vi "Quaternion_Normalize.vi"(11 "Quaternion":T1={"R"=1.0, "V"=[0.0, 0.0, 0.0]}) -> (3 "Normalize":T1={"R"=1.0, "V"=[0.0, 0.0, 0.0]})   [LabVIEW 2019, in "Trajectory_Library.lvlib"]
doc: "Convenience constructors that takes in x and y values directly instead of having to construct a Translation2d.\n\nParameters:\n - X- The x component of the translational component of the pose.\n - Y - The y component of the translational component of the pose.\n - Rotation (Heading) - The rotational component of the pose.\n\nReturns:\n - OUT POSE - Output POSE"
uses:
  QUATERNION.ctl
  Trajectory_Library.lvlib
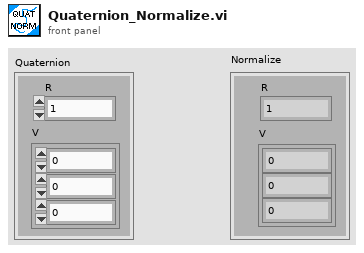
[diagram p1: front panel]
types:
  T1 = typedef "Trajectory_Library.lvlib/QUATERNION.ctl" = cluster{"R":dbl, "V":dbl[]}
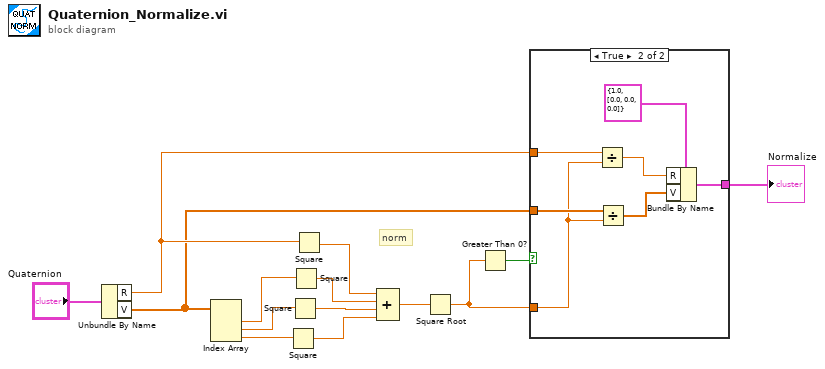
[diagram p0: block diagram]
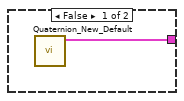
[diagram p2: hidden frame]
diagram:
  # "norm"
  n1 = Unbundle By Name("Quaternion") -> ("R"=w4:dbl, "V"=w3:dbl[])
  n2 = Index Array(array=w3) -> (element #1=w13:dbl, element #2=w12:dbl, element #3=w11:dbl)  [unwired: 3 in]
  n3 = Square(x=w11) -> (x^2=w8:dbl)
  n4 = Square(x=w12) -> (x^2=w9:dbl)
  n5 = Square(x=w13) -> (x^2=w10:dbl)
  n6 = Square(x=w4) -> (x^2=w6:dbl)
  n7 = Compound Arithmetic op=ADD(w6, w10, w9, w8) -> (w7:dbl)
  n8 = Square Root(x=w7) -> (sqrt(x)=w2:dbl)
  n9 = Greater Than 0?(x=w2) -> (x > 0?=w5:bool)
  n10 = case shown="True" w5 {
    tunnel: w4 -> [_ w22]
    tunnel: w3 -> [_ w21]
    tunnel: w2 -> [_ w20]
    tunnel: [w15 w16] -> w1
    frame False {
      n11 = call "Quaternion_New_Default.vi"() -> ("out Quaternion"=w15:T1)  [unwired: 11 in]
    }
    frame True {
      n12 = Divide(x=w22, y=w20) -> (x/y=w18:dbl)
      n13 = Divide(x=w21, y=w20) -> (x/y=w17:dbl[])
      n14 = Bundle By Name(cluster=T1 {"R"=1.0, "V"=[0.0, 0.0, 0.0]} ("sumPOSE"), "R"=w18, "V"=w17) -> (w16:T1)
    }
  }
  "Normalize" <- w1
